vi "Program27.vi"() -> ()   [LabVIEW 2020]
panel:
  out "Wartosc numeryczna":dbl
  out "Jednostka":string
  out "Seperator":string
  out "Parametr":string
  out "Stala czesc komunikatu":string
  out "Polecenie programujące":string
  out "Polecenie z parametrem":string
  in  "Wartość":dbl(knob) scale=0.0..10.0
  in  "Parametr":bool
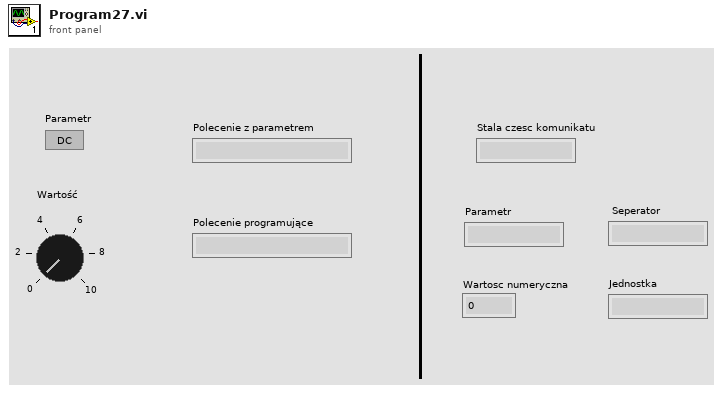
[diagram p1: front panel]
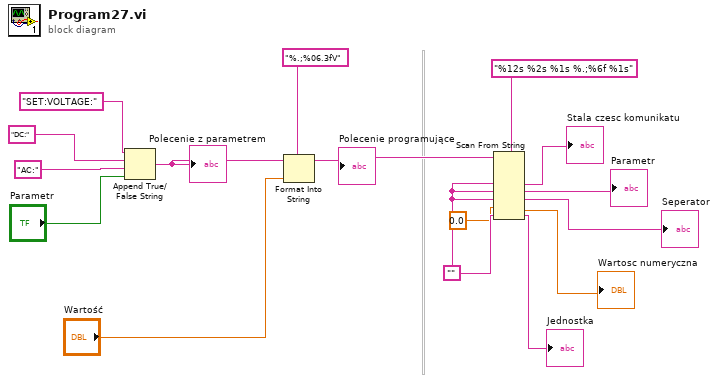
[diagram p0: block diagram]
diagram:
  w3 = ""
  n1 = Append True/False String(1:"Parametr", 2:"AC:", 3:"DC:", 4:"SET:VOLTAGE:") -> (0:w11:string)
  "Polecenie z parametrem" <- w11
  n2 = Format Into String(format string="%.;%06.3fV", initial string=w11, "Wartość") -> (resulting string=w10:string)  [unwired: 1 in, 1 out]
  "Polecenie programujące" <- w10
  n3 = Scan From String(format string="%12s %2s %1s %.;%6f %1s", input string=w10, default 1=w3, default 2=w3, default 3=w3, default 4=0.0, default 5=w3) -> (output 1=→"Stala czesc komunikatu":string, output 2=→"Parametr":string, output 3=→"Seperator":string, output 4=→"Wartosc numeryczna":dbl, output 5=→"Jednostka":string)  [unwired: 2 in, 3 out]
